vi "Bildwechsel.vi"(5 "Referenz Permanent":refnum<vi>, 7 "Referenz Mitte":refnum<vi>, 8 "nächstes Bild":T1=enum."Grafik") -> (1 "aktuelle Bildnummer":T1=enum."Grafik", 3 "VI-Referenz neu":refnum<vi>)   [LabVIEW 2020, in "Bildwechsel.lvlib"]
uses:
  Bildwechsel.lvlib
  Bild-Auswahl.ctl
  <vilib>/Utility/miscctls.llb/LVBoundsTypeDef.ctl
  VisBx Anzeige.vi
  EPA 1065/Dichtheitstest 1065-345/Konfig Leak Check.vi
  EPA 1065/Gas Analyzer Drift 1065-550/Drift Verification Konfig.vi
  EPA 1065/Interference verificaton 1065-366/VI Interference Konfig.vi
  EPA 1065/T90 1065-308/T90 Test Konfig.vi
  EPA 1065/Interference verificaton 1065-375/VI Interference Konfig.vi
  VI Anlagengrenzwerte Amium PNS.vi
  Seiten/EL3000/FID/VI FID Konfig.vi
  Seiten/EL3000/PMA/VI PMA Konfig.vi
  VI Konfiguration Kalibriergase.vi
  Seiten/Lambdasonde/VI Konfig LAMBDA.vi
  Schedule Modul/VI Schedule Seite.vi
  Seiten/System Einstellungen V2/System und Gaseinstellung V2.vi
  Seiten/CAN Konfig/VI CAN Konfig.vi
  EPA 1065/HovaCAL Interference verification/VI Interference Konfig.vi
  Allgemein/allgemeine Sub-VIs.lvlib
  Seiten/Grafik/Grafik.lvlib
  Seiten/Anlagengrenzwerte/Anlagengrenzwerte.lvlib
  Seiten/Gaszuordnung AO/Gaszuordnung AO.lvlib
  Seiten/Erweiterte Konfig/Erweiterte Konfig.lvlib
  Seiten/Anlagenuebersicht/VisBx Anzeige/Anlagenuebersicht.lvlib
  Seiten/FT-IR/FT-IR.lvlib
  PNS/PNS.lvlib
  Stoerungen/Stoerungen.lvlib
  Seiten/Statusuebersicht/Statusuebersicht.lvlib
  Seiten/EL3000/FID/FID.lvlib
  Seiten/EL3000/PMA/PMA.lvlib
  Seiten/CalGas Aufschaltung/CalGas Aufschaltung.lvlib
  Seiten/Lambdasonde/Lambda_ Komm.lvlib
  Amium PNS/Amium PNS.lvlib
  Linearisierung V2/Linearisierung v2.lvlib
  EPA 1065/Dichtheitstest 1065-345/Dichtheitstest 1065-345.lvlib
  EPA 1065/T90 1065-308/T90 Test 1065-308.lvlib
  EPA 1065/ANR Test 1065-305/ARN Test 1065-305.lvlib
  EPA 1065/Interference verificaton 1065-375/Interference verificaton 1065-375.lvlib
  EPA 1065/Interference verificaton 1065-366/Interference verificaton 1065-366.lvlib
  Schedule Modul/Schedule Modul.lvlib
  Seiten/Log Konfig/LogKonfig.lvlib
  Seiten/System Einstellungen V2/System Einstellungen V2.lvlib
  EPA 1065/Gas Analyzer Drift 1065-550/Gas Analyzer Drift 1065-550.lvlib
  Seiten/CAN Konfig/CAN Konfig.lvlib
  EPA 1065/HovaCAL Interference verification/HovaCAL Interference verificaton.lvlib
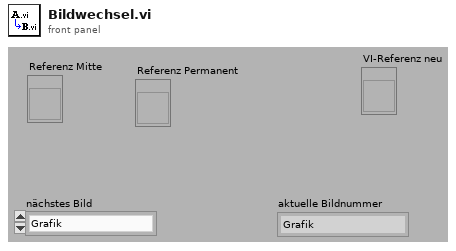
[diagram p1: front panel]
types:
  T1 = typedef "Bildwechsel.lvlib/Bild-Auswahl.ctl" = enum16{"lesen", "Initialisieren", "Beenden", "Grafik", "Anlagenübersicht", "Anlagengrenzwerte", "Log Konfig", "Gaszuordnung AO", "Erw. Konfiguration", "FT-IR  ", "Störmeldungen", "Störmeldepuffer", "Störmeldekonfig", "PNS Grenzwerte", "Statusübersicht", "Linearisierung", "ARN", "EPA Dichtheitstest", "FID", "PMA", "CalGas", "Lambda", "Interference", "Amium PNS", "EPA T90", "Interference N2O", "Scheduler", "Systemeinstellungen", "EPA Drift", "CAN Konfig", "HovaCAL Interference"}
  T2 = typedef "LVBoundsTypeDef.ctl" = cluster{"Width":u32, "Height":u32}
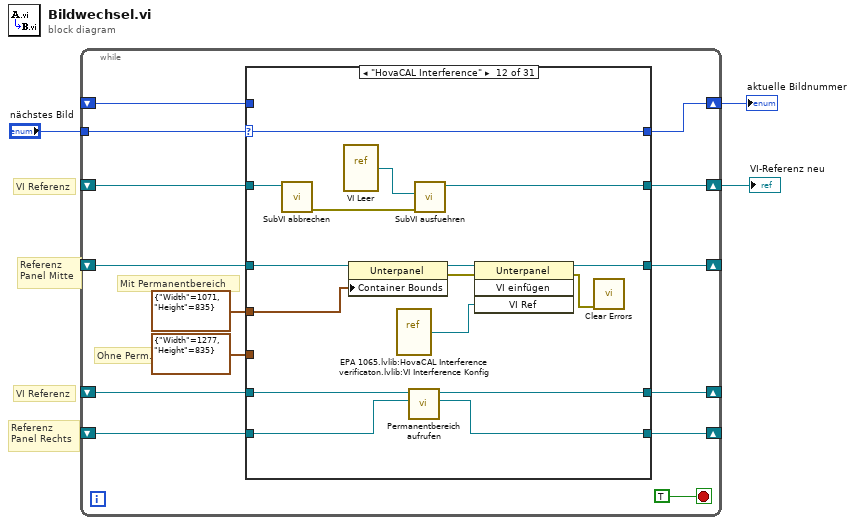
[diagram p0: block diagram]
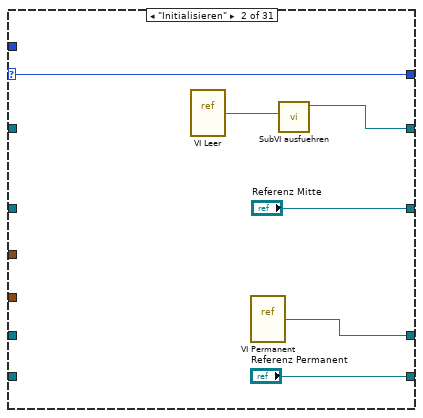
[diagram p3: hidden frame]
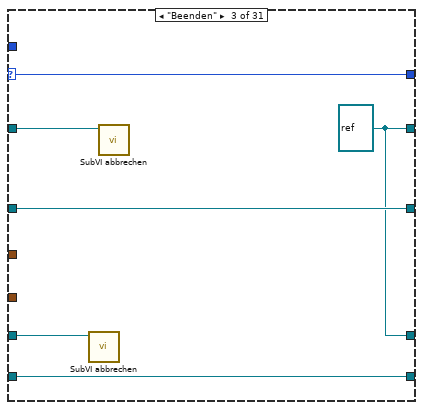
[diagram p4: hidden frame]
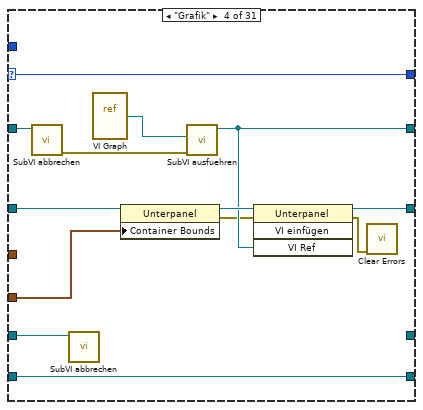
[diagram p5: hidden frame]
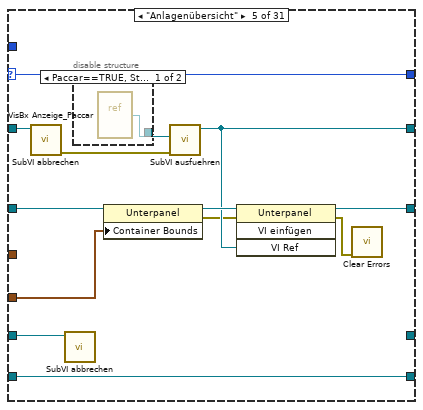
[diagram p6: hidden frame]
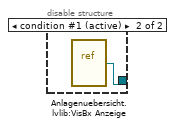
[diagram p7: hidden frame]
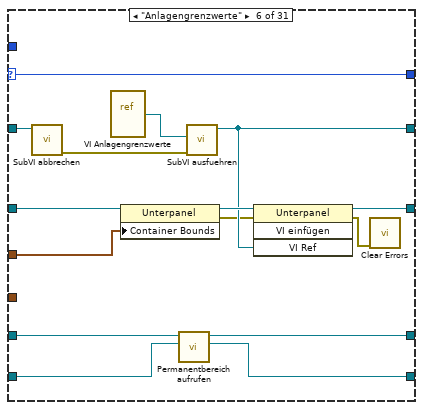
[diagram p8: hidden frame]
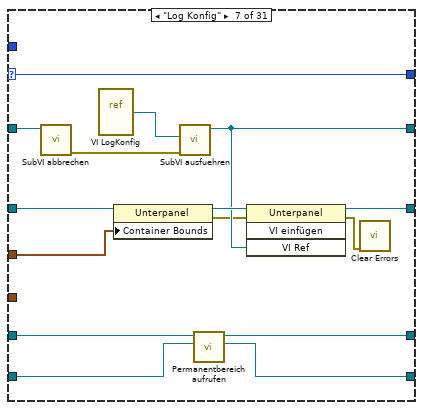
[diagram p9: hidden frame]
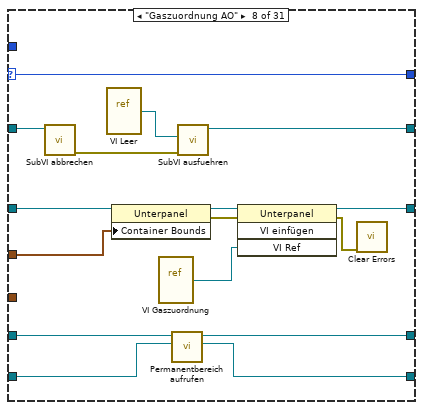
[diagram p10: hidden frame]
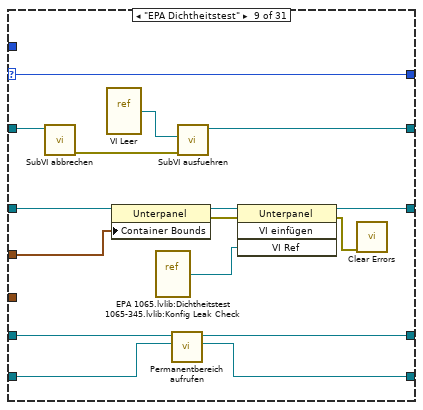
[diagram p11: hidden frame]
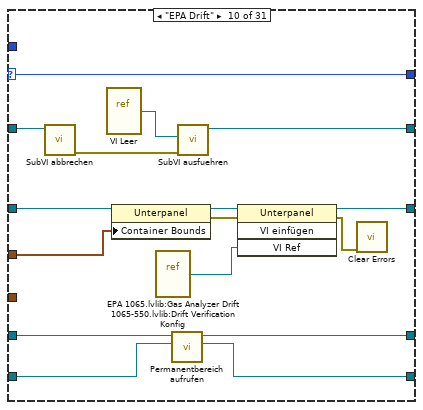
[diagram p12: hidden frame]
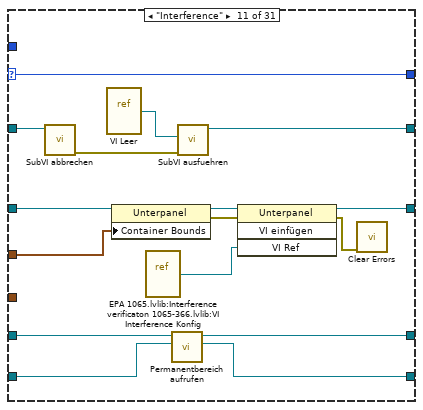
[diagram p13: hidden frame]
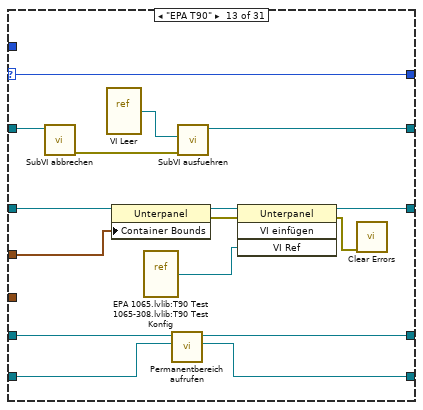
[diagram p14: hidden frame]
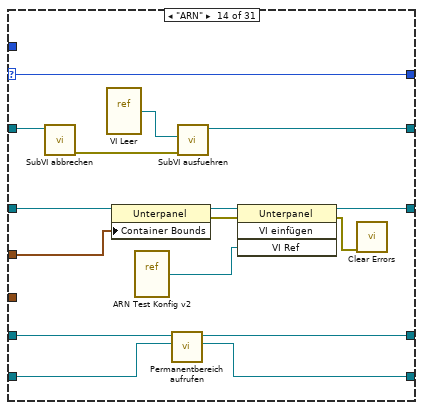
[diagram p15: hidden frame]
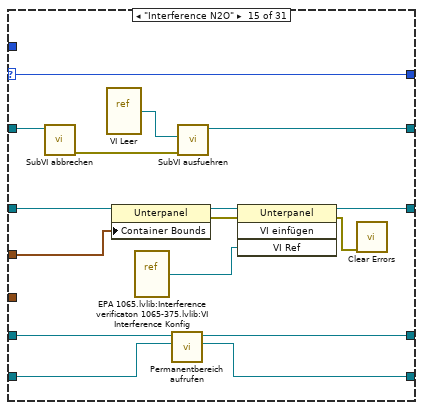
[diagram p16: hidden frame]
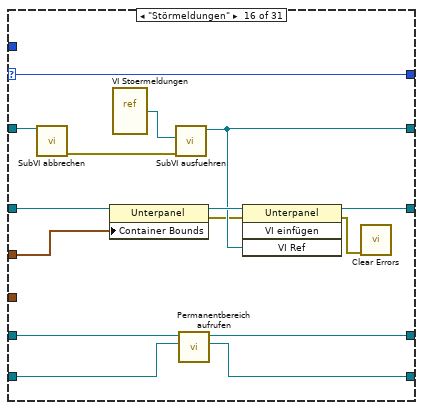
[diagram p17: hidden frame]
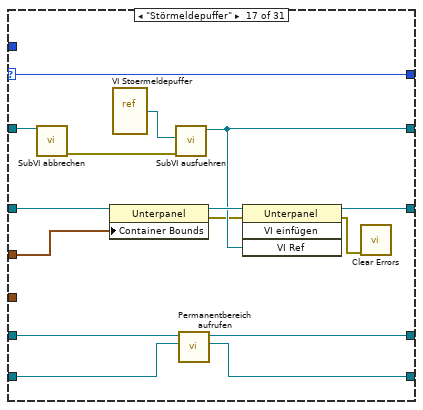
[diagram p18: hidden frame]
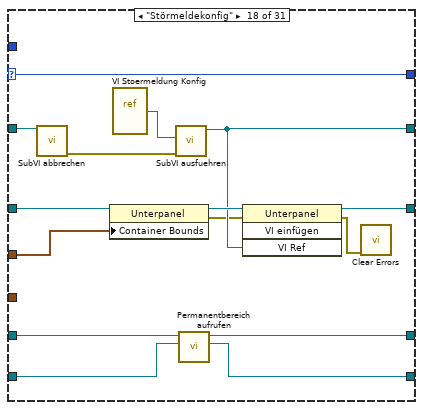
[diagram p19: hidden frame]
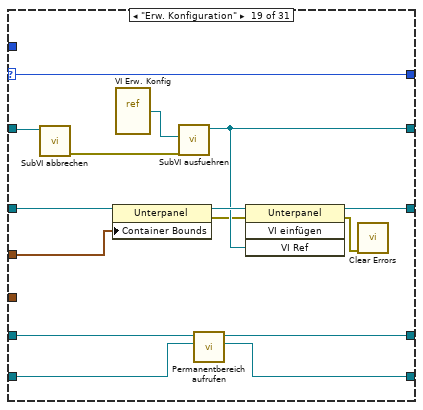
[diagram p20: hidden frame]
diagram:
  # "VI Referenz"
  # "VI Referenz"
  # "Referenz\nPanel Rechts"
  # "Referenz\nPanel Mitte"
  n1 = while {
    shift-right: [w15] -> w2
    shift-left: _ -> [w14]
    tunnel: "nächstes Bild" -> [w13]
    shift-right: [w12] -> _
    shift-left: _ -> [w11]
    shift-right: [w9] -> _
    shift-left: _ -> [w8]
    shift-right: [w7] -> w1
    shift-left: _ -> [w6]
    shift-right: [w5] -> _
    shift-left: _ -> [w4]
    stop <- TRUE stop-if-true
    # "Ohne Perm."
    # "Mit Permanentbereich"
    n2 = case shown="\"HovaCAL Interference\"" w13 {
      selector: w13 -> [_ w25 w32 w41 w53 w70 w85 w100 w117 w133 w149 w165 w181 w197 w213 w228 w243 w258 w273 w289 w304 w319 w334 w349 w364 w379 w394 w411 w427 w442 w457]
      tunnel: w14 -> [w21 _ w34 w46 w59 w76 w89 w106 w122 w138 w154 w170 w186 w202 w218 w231 w246 w261 w279 w294 w309 w324 w339 w354 w369 w384 w399 w415 w418 w433 w448]
      tunnel: [w21 w27 w31 w45 w58 w75 w91 w104 w120 w136 w152 w168 w184 w200 w216 w233 w248 w263 w278 w293 w308 w323 w338 w353 w368 w383 w398 w414 w426 w441 w456] -> w15
      tunnel: w11 -> [w20 _ w33 w44 w57 w74 w90 w107 w123 w139 w155 w171 w187 w203 w219 w232 w247 w262 w277 w292 w307 w322 w337 w352 w367 w382 w397 w413 w424 w439 w454]
      tunnel: T2 {"Width"=1071, "Height"=835} ("groß") -> [_ _ _ _ _ w73 w88 w105 w121 w137 w153 w169 w185 w201 w217 w229 w244 w259 w276 w288 w303 w318 w333 w348 w363 w378 w393 w410 w419 w434 w449]
      tunnel: T2 {"Width"=1277, "Height"=835} ("groß") -> [_ _ _ w40 w56 _ _ _ _ _ _ _ _ _ _ _ _ _ _ _ _ _ _ _ _ _ _ _ _ _ _]
      tunnel: [w20 "Referenz Mitte" w33 w42 w54 w71 w86 w103 w119 w135 w151 w167 w183 w199 w215 w230 w245 w260 w274 w290 w305 w320 w335 w350 w365 w380 w395 w412 w425 w440 w455] -> w12
      tunnel: [w19 w23 w31 _ _ w68 w81 w97 w114 w130 w146 w162 w178 w194 w210 w226 w241 w256 w269 w286 w301 w316 w331 w346 w361 w376 w391 w408 w421 w436 w451] -> w9
      tunnel: w8 -> [w19 _ w29 w39 w51 w69 w82 w98 w115 w131 w147 w163 w179 w195 w211 w227 w242 w257 w270 w287 w302 w317 w332 w347 w362 w377 w392 w409 w423 w438 w453]
      tunnel: [w22 w25 w32 w41 w53 w70 w85 w100 w117 w133 w149 w165 w181 w197 w213 w228 w243 w258 w273 w289 w304 w319 w334 w349 w364 w379 w394 w411 w427 w442 w457] -> w7
      tunnel: w6 -> [w22 _ _ _ _ _ _ _ _ _ _ _ _ _ _ _ _ _ _ _ _ _ _ _ _ _ _ _ _ _ _]
      tunnel: [w18 "Referenz Permanent" w30 w38 w50 w66 w79 w95 w112 w128 w144 w160 w176 w192 w208 w225 w240 w255 w268 w284 w299 w314 w329 w344 w359 w374 w389 w406 w420 w435 w450] -> w5
      tunnel: w4 -> [w18 _ w30 w38 w50 w67 w80 w96 w113 w129 w145 w161 w177 w193 w209 w224 w239 w254 w267 w285 w300 w315 w330 w345 w360 w375 w390 w407 w422 w437 w452]
      frame "lesen" {
      }
      frame "Initialisieren" {
        n3 = vi-ref "VI Leer.vi"() -> (w26:refnum<vi>)
        n4 = vi-ref "VI Permanent.vi"() -> (w23:refnum<vi>)
        n5 = call "SubVI ausfuehren.vi"("Referenz"=w26) -> ("vi reference"=w27:refnum<vi>)  [unwired: 10 in]
      }
      frame "Beenden" {
        w31 = refnum<vi> refnum ("vi reference")
        n6 = call "SubVI abbrechen.vi"("vi reference"=w29) -> ()  [unwired: 1 in, 6 out]
        n7 = call "SubVI abbrechen.vi"("vi reference"=w34) -> ()  [unwired: 1 in, 6 out]
      }
      frame "Grafik" {
        n8 = call "SubVI abbrechen.vi"("vi reference"=w46) -> ("error out"=w35:errorcluster)  [unwired: 1 in, 5 out]
        n9 = call "SubVI abbrechen.vi"("vi reference"=w39) -> ()  [unwired: 1 in, 6 out]
        n10 = vi-ref "VI Graph.vi"() -> (w43:refnum<vi>)
        n11 = property on="Eigenschaftsknoten" class="Unterpanel"(reference=w44, "Container Bounds"=w40) -> (reference out=w47:refnum<vi>, error out=w37:errorcluster)  [unwired: 1 in]
        n12 = call "SubVI ausfuehren.vi"("Fehler"=w35, "Referenz"=w43) -> ("vi reference"=w45:refnum<vi>)  [unwired: 9 in]
        n13 = invoke on="Methodenknoten" class="Unterpanel" method="VI einfügen"(reference=w47, error in=w37, "VI Ref"=w45) -> (reference out=w42:refnum<vi>, error out=w36:errorcluster)  [unwired: 1 in, 2 out]
        n14 = call <vilib>:"Clear Errors.vi"("error in (no error)"=w36) -> ()  [unwired: 5 in, 2 out]
      }
      frame "Anlagenübersicht" {
        n15 = call "SubVI abbrechen.vi"("vi reference"=w59) -> ("error out"=w48:errorcluster)  [unwired: 1 in, 5 out]
        n16 = call "SubVI abbrechen.vi"("vi reference"=w51) -> ()  [unwired: 1 in, 6 out]
        n17 = disable-structure shown="Paccar==TRUE, Standard" {
          disable-tunnel: [w61 w62] -> w55
          frame condition #0 {
            n18 = vi-ref "VisBx Anzeige_Paccar.vi"() -> (w61:refnum<vi>)
          }
          frame condition #1 (active) {
            n19 = vi-ref "Anlagenuebersicht.lvlib:VisBx Anzeige.vi"() -> (w62:refnum<vi>)
          }
        }
        n20 = property on="Eigenschaftsknoten" class="Unterpanel"(reference=w57, "Container Bounds"=w56) -> (reference out=w60:refnum<vi>, error out=w52:errorcluster)  [unwired: 1 in]
        n21 = call "SubVI ausfuehren.vi"("Fehler"=w48, "Referenz"=w55) -> ("vi reference"=w58:refnum<vi>)  [unwired: 9 in]
        n22 = invoke on="Methodenknoten" class="Unterpanel" method="VI einfügen"(reference=w60, error in=w52, "VI Ref"=w58) -> (reference out=w54:refnum<vi>, error out=w49:errorcluster)  [unwired: 1 in, 2 out]
        n23 = call <vilib>:"Clear Errors.vi"("error in (no error)"=w49) -> ()  [unwired: 5 in, 2 out]
      }
      frame "Anlagengrenzwerte" {
        n24 = call "SubVI abbrechen.vi"("vi reference"=w76) -> ("error out"=w63:errorcluster)  [unwired: 1 in, 5 out]
        n25 = vi-ref "VI Anlagengrenzwerte.vi"() -> (w72:refnum<vi>)
        n26 = property on="Eigenschaftsknoten" class="Unterpanel"(reference=w74, "Container Bounds"=w73) -> (reference out=w77:refnum<vi>, error out=w65:errorcluster)  [unwired: 1 in]
        n27 = call "Permanentbereich aufrufen.vi"("Permanent (Eingang)"=w67, "VI (Eingang)"=w69) -> ("Permanent (Ausgang)"=w66:refnum<vi>, "VI (Ausgang)"=w68:refnum<vi>)  [unwired: 8 in]
        n28 = call "SubVI ausfuehren.vi"("Fehler"=w63, "Referenz"=w72) -> ("vi reference"=w75:refnum<vi>)  [unwired: 9 in]
        n29 = invoke on="Methodenknoten" class="Unterpanel" method="VI einfügen"(reference=w77, error in=w65, "VI Ref"=w75) -> (reference out=w71:refnum<vi>, error out=w64:errorcluster)  [unwired: 1 in, 2 out]
        n30 = call <vilib>:"Clear Errors.vi"("error in (no error)"=w64) -> ()  [unwired: 5 in, 2 out]
      }
      frame "Log Konfig" {
        n31 = call "SubVI abbrechen.vi"("vi reference"=w89) -> ("error out"=w78:errorcluster)  [unwired: 1 in, 5 out]
        n32 = vi-ref "VI LogKonfig.vi"() -> (w87:refnum<vi>)
        n33 = property on="Eigenschaftsknoten" class="Unterpanel"(reference=w90, "Container Bounds"=w88) -> (reference out=w92:refnum<vi>, error out=w84:errorcluster)  [unwired: 1 in]
        n34 = call "SubVI ausfuehren.vi"("Fehler"=w78, "Referenz"=w87) -> ("vi reference"=w91:refnum<vi>)  [unwired: 9 in]
        n35 = call "Permanentbereich aufrufen.vi"("Permanent (Eingang)"=w80, "VI (Eingang)"=w82) -> ("Permanent (Ausgang)"=w79:refnum<vi>, "VI (Ausgang)"=w81:refnum<vi>)  [unwired: 8 in]
        n36 = invoke on="Methodenknoten" class="Unterpanel" method="VI einfügen"(reference=w92, error in=w84, "VI Ref"=w91) -> (reference out=w86:refnum<vi>, error out=w83:errorcluster)  [unwired: 1 in, 2 out]
        n37 = call <vilib>:"Clear Errors.vi"("error in (no error)"=w83) -> ()  [unwired: 5 in, 2 out]
      }
      frame "Gaszuordnung AO" {
        n38 = call "SubVI abbrechen.vi"("vi reference"=w106) -> ("error out"=w93:errorcluster)  [unwired: 1 in, 5 out]
        n39 = vi-ref "VI Leer.vi"() -> (w102:refnum<vi>)
        n40 = property on="Eigenschaftsknoten" class="Unterpanel"(reference=w107, "Container Bounds"=w105) -> (reference out=w108:refnum<vi>, error out=w94:errorcluster)  [unwired: 1 in]
        n41 = vi-ref "VI Gaszuordnung.vi"() -> (w101:refnum<vi>)
        n42 = call "Permanentbereich aufrufen.vi"("Permanent (Eingang)"=w96, "VI (Eingang)"=w98) -> ("Permanent (Ausgang)"=w95:refnum<vi>, "VI (Ausgang)"=w97:refnum<vi>)  [unwired: 8 in]
        n43 = call "SubVI ausfuehren.vi"("Fehler"=w93, "Referenz"=w102) -> ("vi reference"=w104:refnum<vi>)  [unwired: 9 in]
        n44 = invoke on="Methodenknoten" class="Unterpanel" method="VI einfügen"(reference=w108, error in=w94, "VI Ref"=w101) -> (reference out=w103:refnum<vi>, error out=w99:errorcluster)  [unwired: 1 in, 2 out]
        n45 = call <vilib>:"Clear Errors.vi"("error in (no error)"=w99) -> ()  [unwired: 5 in, 2 out]
      }
      frame "EPA Dichtheitstest" {
        n46 = call "SubVI abbrechen.vi"("vi reference"=w122) -> ("error out"=w110:errorcluster)  [unwired: 1 in, 5 out]
        n47 = vi-ref "VI Leer.vi"() -> (w118:refnum<vi>)
        n48 = property on="Eigenschaftsknoten" class="Unterpanel"(reference=w123, "Container Bounds"=w121) -> (reference out=w124:refnum<vi>, error out=w111:errorcluster)  [unwired: 1 in]
        n49 = vi-ref "EPA 1065.lvlib:Dichtheitstest 1065-345.lvlib:Konfig Leak Check.vi"() -> (w109:refnum<vi>)
        n50 = call "Permanentbereich aufrufen.vi"("Permanent (Eingang)"=w113, "VI (Eingang)"=w115) -> ("Permanent (Ausgang)"=w112:refnum<vi>, "VI (Ausgang)"=w114:refnum<vi>)  [unwired: 8 in]
        n51 = call "SubVI ausfuehren.vi"("Fehler"=w110, "Referenz"=w118) -> ("vi reference"=w120:refnum<vi>)  [unwired: 9 in]
        n52 = invoke on="Methodenknoten" class="Unterpanel" method="VI einfügen"(reference=w124, error in=w111, "VI Ref"=w109) -> (reference out=w119:refnum<vi>, error out=w116:errorcluster)  [unwired: 1 in, 2 out]
        n53 = call <vilib>:"Clear Errors.vi"("error in (no error)"=w116) -> ()  [unwired: 5 in, 2 out]
      }
      frame "EPA Drift" {
        n54 = call "SubVI abbrechen.vi"("vi reference"=w138) -> ("error out"=w126:errorcluster)  [unwired: 1 in, 5 out]
        n55 = vi-ref "VI Leer.vi"() -> (w134:refnum<vi>)
        n56 = property on="Eigenschaftsknoten" class="Unterpanel"(reference=w139, "Container Bounds"=w137) -> (reference out=w140:refnum<vi>, error out=w127:errorcluster)  [unwired: 1 in]
        n57 = vi-ref "EPA 1065.lvlib:Gas Analyzer Drift 1065-550.lvlib:Drift Verification Konfig.vi"() -> (w125:refnum<vi>)
        n58 = call "Permanentbereich aufrufen.vi"("Permanent (Eingang)"=w129, "VI (Eingang)"=w131) -> ("Permanent (Ausgang)"=w128:refnum<vi>, "VI (Ausgang)"=w130:refnum<vi>)  [unwired: 8 in]
        n59 = call "SubVI ausfuehren.vi"("Fehler"=w126, "Referenz"=w134) -> ("vi reference"=w136:refnum<vi>)  [unwired: 9 in]
        n60 = invoke on="Methodenknoten" class="Unterpanel" method="VI einfügen"(reference=w140, error in=w127, "VI Ref"=w125) -> (reference out=w135:refnum<vi>, error out=w132:errorcluster)  [unwired: 1 in, 2 out]
        n61 = call <vilib>:"Clear Errors.vi"("error in (no error)"=w132) -> ()  [unwired: 5 in, 2 out]
      }
      frame "Interference" {
        n62 = call "SubVI abbrechen.vi"("vi reference"=w154) -> ("error out"=w142:errorcluster)  [unwired: 1 in, 5 out]
        n63 = vi-ref "VI Leer.vi"() -> (w150:refnum<vi>)
        n64 = property on="Eigenschaftsknoten" class="Unterpanel"(reference=w155, "Container Bounds"=w153) -> (reference out=w156:refnum<vi>, error out=w143:errorcluster)  [unwired: 1 in]
        n65 = vi-ref "EPA 1065.lvlib:Interference verificaton 1065-366.lvlib:VI Interference Konfig.vi"() -> (w141:refnum<vi>)
        n66 = call "Permanentbereich aufrufen.vi"("Permanent (Eingang)"=w145, "VI (Eingang)"=w147) -> ("Permanent (Ausgang)"=w144:refnum<vi>, "VI (Ausgang)"=w146:refnum<vi>)  [unwired: 8 in]
        n67 = call "SubVI ausfuehren.vi"("Fehler"=w142, "Referenz"=w150) -> ("vi reference"=w152:refnum<vi>)  [unwired: 9 in]
        n68 = invoke on="Methodenknoten" class="Unterpanel" method="VI einfügen"(reference=w156, error in=w143, "VI Ref"=w141) -> (reference out=w151:refnum<vi>, error out=w148:errorcluster)  [unwired: 1 in, 2 out]
        n69 = call <vilib>:"Clear Errors.vi"("error in (no error)"=w148) -> ()  [unwired: 5 in, 2 out]
      }
      frame "HovaCAL Interference" {
        n70 = call "SubVI abbrechen.vi"("vi reference"=w170) -> ("error out"=w158:errorcluster)  [unwired: 1 in, 5 out]
        n71 = vi-ref "VI Leer.vi"() -> (w166:refnum<vi>)
        n72 = property on="Eigenschaftsknoten" class="Unterpanel"(reference=w171, "Container Bounds"=w169) -> (reference out=w172:refnum<vi>, error out=w159:errorcluster)  [unwired: 1 in]
        n73 = vi-ref "EPA 1065.lvlib:HovaCAL Interference verificaton.lvlib:VI Interference Konfig.vi"() -> (w157:refnum<vi>)
        n74 = call "Permanentbereich aufrufen.vi"("Permanent (Eingang)"=w161, "VI (Eingang)"=w163) -> ("Permanent (Ausgang)"=w160:refnum<vi>, "VI (Ausgang)"=w162:refnum<vi>)  [unwired: 8 in]
        n75 = call "SubVI ausfuehren.vi"("Fehler"=w158, "Referenz"=w166) -> ("vi reference"=w168:refnum<vi>)  [unwired: 9 in]
        n76 = invoke on="Methodenknoten" class="Unterpanel" method="VI einfügen"(reference=w172, error in=w159, "VI Ref"=w157) -> (reference out=w167:refnum<vi>, error out=w164:errorcluster)  [unwired: 1 in, 2 out]
        n77 = call <vilib>:"Clear Errors.vi"("error in (no error)"=w164) -> ()  [unwired: 5 in, 2 out]
      }
      frame "EPA T90" {
        n78 = call "SubVI abbrechen.vi"("vi reference"=w186) -> ("error out"=w174:errorcluster)  [unwired: 1 in, 5 out]
        n79 = vi-ref "VI Leer.vi"() -> (w182:refnum<vi>)
        n80 = property on="Eigenschaftsknoten" class="Unterpanel"(reference=w187, "Container Bounds"=w185) -> (reference out=w188:refnum<vi>, error out=w175:errorcluster)  [unwired: 1 in]
        n81 = vi-ref "EPA 1065.lvlib:T90 Test 1065-308.lvlib:T90 Test Konfig.vi"() -> (w173:refnum<vi>)
        n82 = call "Permanentbereich aufrufen.vi"("Permanent (Eingang)"=w177, "VI (Eingang)"=w179) -> ("Permanent (Ausgang)"=w176:refnum<vi>, "VI (Ausgang)"=w178:refnum<vi>)  [unwired: 8 in]
        n83 = call "SubVI ausfuehren.vi"("Fehler"=w174, "Referenz"=w182) -> ("vi reference"=w184:refnum<vi>)  [unwired: 9 in]
        n84 = invoke on="Methodenknoten" class="Unterpanel" method="VI einfügen"(reference=w188, error in=w175, "VI Ref"=w173) -> (reference out=w183:refnum<vi>, error out=w180:errorcluster)  [unwired: 1 in, 2 out]
        n85 = call <vilib>:"Clear Errors.vi"("error in (no error)"=w180) -> ()  [unwired: 5 in, 2 out]
      }
      frame "ARN" {
        n86 = call "SubVI abbrechen.vi"("vi reference"=w202) -> ("error out"=w190:errorcluster)  [unwired: 1 in, 5 out]
        n87 = vi-ref "VI Leer.vi"() -> (w198:refnum<vi>)
        n88 = property on="Eigenschaftsknoten" class="Unterpanel"(reference=w203, "Container Bounds"=w201) -> (reference out=w204:refnum<vi>, error out=w191:errorcluster)  [unwired: 1 in]
        n89 = vi-ref "ARN Test Konfig v2.vi"() -> (w189:refnum<vi>)
        n90 = call "Permanentbereich aufrufen.vi"("Permanent (Eingang)"=w193, "VI (Eingang)"=w195) -> ("Permanent (Ausgang)"=w192:refnum<vi>, "VI (Ausgang)"=w194:refnum<vi>)  [unwired: 8 in]
        n91 = call "SubVI ausfuehren.vi"("Fehler"=w190, "Referenz"=w198) -> ("vi reference"=w200:refnum<vi>)  [unwired: 9 in]
        n92 = invoke on="Methodenknoten" class="Unterpanel" method="VI einfügen"(reference=w204, error in=w191, "VI Ref"=w189) -> (reference out=w199:refnum<vi>, error out=w196:errorcluster)  [unwired: 1 in, 2 out]
        n93 = call <vilib>:"Clear Errors.vi"("error in (no error)"=w196) -> ()  [unwired: 5 in, 2 out]
      }
      frame "Interference N2O" {
        n94 = call "SubVI abbrechen.vi"("vi reference"=w218) -> ("error out"=w206:errorcluster)  [unwired: 1 in, 5 out]
        n95 = vi-ref "VI Leer.vi"() -> (w214:refnum<vi>)
        n96 = property on="Eigenschaftsknoten" class="Unterpanel"(reference=w219, "Container Bounds"=w217) -> (reference out=w220:refnum<vi>, error out=w207:errorcluster)  [unwired: 1 in]
        n97 = vi-ref "EPA 1065.lvlib:Interference verificaton 1065-375.lvlib:VI Interference Konfig.vi"() -> (w205:refnum<vi>)
        n98 = call "Permanentbereich aufrufen.vi"("Permanent (Eingang)"=w209, "VI (Eingang)"=w211) -> ("Permanent (Ausgang)"=w208:refnum<vi>, "VI (Ausgang)"=w210:refnum<vi>)  [unwired: 8 in]
        n99 = call "SubVI ausfuehren.vi"("Fehler"=w206, "Referenz"=w214) -> ("vi reference"=w216:refnum<vi>)  [unwired: 9 in]
        n100 = invoke on="Methodenknoten" class="Unterpanel" method="VI einfügen"(reference=w220, error in=w207, "VI Ref"=w205) -> (reference out=w215:refnum<vi>, error out=w212:errorcluster)  [unwired: 1 in, 2 out]
        n101 = call <vilib>:"Clear Errors.vi"("error in (no error)"=w212) -> ()  [unwired: 5 in, 2 out]
      }
      frame "Störmeldungen" {
        n102 = call "SubVI abbrechen.vi"("vi reference"=w231) -> ("error out"=w221:errorcluster)  [unwired: 1 in, 5 out]
        n103 = property on="Eigenschaftsknoten" class="Unterpanel"(reference=w232, "Container Bounds"=w229) -> (reference out=w235:refnum<vi>, error out=w223:errorcluster)  [unwired: 1 in]
        n104 = vi-ref "VI Stoermeldungen.vi"() -> (w234:refnum<vi>)
        n105 = call "SubVI ausfuehren.vi"("Fehler"=w221, "Referenz"=w234) -> ("vi reference"=w233:refnum<vi>)  [unwired: 9 in]
        n106 = call "Permanentbereich aufrufen.vi"("Permanent (Eingang)"=w224, "VI (Eingang)"=w227) -> ("Permanent (Ausgang)"=w225:refnum<vi>, "VI (Ausgang)"=w226:refnum<vi>)  [unwired: 8 in]
        n107 = invoke on="Methodenknoten" class="Unterpanel" method="VI einfügen"(reference=w235, error in=w223, "VI Ref"=w233) -> (reference out=w230:refnum<vi>, error out=w222:errorcluster)  [unwired: 1 in, 2 out]
        n108 = call <vilib>:"Clear Errors.vi"("error in (no error)"=w222) -> ()  [unwired: 5 in, 2 out]
      }
      frame "Störmeldepuffer" {
        n109 = call "SubVI abbrechen.vi"("vi reference"=w246) -> ("error out"=w236:errorcluster)  [unwired: 1 in, 5 out]
        n110 = property on="Eigenschaftsknoten" class="Unterpanel"(reference=w247, "Container Bounds"=w244) -> (reference out=w250:refnum<vi>, error out=w238:errorcluster)  [unwired: 1 in]
        n111 = vi-ref "VI Stoermeldepuffer.vi"() -> (w249:refnum<vi>)
        n112 = call "SubVI ausfuehren.vi"("Fehler"=w236, "Referenz"=w249) -> ("vi reference"=w248:refnum<vi>)  [unwired: 9 in]
        n113 = call "Permanentbereich aufrufen.vi"("Permanent (Eingang)"=w239, "VI (Eingang)"=w242) -> ("Permanent (Ausgang)"=w240:refnum<vi>, "VI (Ausgang)"=w241:refnum<vi>)  [unwired: 8 in]
        n114 = invoke on="Methodenknoten" class="Unterpanel" method="VI einfügen"(reference=w250, error in=w238, "VI Ref"=w248) -> (reference out=w245:refnum<vi>, error out=w237:errorcluster)  [unwired: 1 in, 2 out]
        n115 = call <vilib>:"Clear Errors.vi"("error in (no error)"=w237) -> ()  [unwired: 5 in, 2 out]
      }
      frame "Störmeldekonfig" {
        n116 = call "SubVI abbrechen.vi"("vi reference"=w261) -> ("error out"=w251:errorcluster)  [unwired: 1 in, 5 out]
        n117 = property on="Eigenschaftsknoten" class="Unterpanel"(reference=w262, "Container Bounds"=w259) -> (reference out=w265:refnum<vi>, error out=w253:errorcluster)  [unwired: 1 in]
        n118 = vi-ref "VI Stoermeldung Konfig.vi"() -> (w264:refnum<vi>)
        n119 = call "SubVI ausfuehren.vi"("Fehler"=w251, "Referenz"=w264) -> ("vi reference"=w263:refnum<vi>)  [unwired: 9 in]
        n120 = call "Permanentbereich aufrufen.vi"("Permanent (Eingang)"=w254, "VI (Eingang)"=w257) -> ("Permanent (Ausgang)"=w255:refnum<vi>, "VI (Ausgang)"=w256:refnum<vi>)  [unwired: 8 in]
        n121 = invoke on="Methodenknoten" class="Unterpanel" method="VI einfügen"(reference=w265, error in=w253, "VI Ref"=w263) -> (reference out=w260:refnum<vi>, error out=w252:errorcluster)  [unwired: 1 in, 2 out]
        n122 = call <vilib>:"Clear Errors.vi"("error in (no error)"=w252) -> ()  [unwired: 5 in, 2 out]
      }
      frame "Erw. Konfiguration" {
        n123 = call "SubVI abbrechen.vi"("vi reference"=w279) -> ("error out"=w266:errorcluster)  [unwired: 1 in, 5 out]
        n124 = property on="Eigenschaftsknoten" class="Unterpanel"(reference=w277, "Container Bounds"=w276) -> (reference out=w280:refnum<vi>, error out=w272:errorcluster)  [unwired: 1 in]
        n125 = vi-ref "VI Erw. Konfig.vi"() -> (w275:refnum<vi>)
        n126 = call "SubVI ausfuehren.vi"("Fehler"=w266, "Referenz"=w275) -> ("vi reference"=w278:refnum<vi>)  [unwired: 9 in]
        n127 = call "Permanentbereich aufrufen.vi"("Permanent (Eingang)"=w267, "VI (Eingang)"=w270) -> ("Permanent (Ausgang)"=w268:refnum<vi>, "VI (Ausgang)"=w269:refnum<vi>)  [unwired: 8 in]
        n128 = invoke on="Methodenknoten" class="Unterpanel" method="VI einfügen"(reference=w280, error in=w272, "VI Ref"=w278) -> (reference out=w274:refnum<vi>, error out=w271:errorcluster)  [unwired: 1 in, 2 out]
        n129 = call <vilib>:"Clear Errors.vi"("error in (no error)"=w271) -> ()  [unwired: 5 in, 2 out]
      }
      frame "FT-IR  " {
        n130 = call "SubVI abbrechen.vi"("vi reference"=w294) -> ("error out"=w281:errorcluster)  [unwired: 1 in, 5 out]
        n131 = vi-ref "VI Konfig FT-IR.vi"() -> (w291:refnum<vi>)
        n132 = property on="Eigenschaftsknoten" class="Unterpanel"(reference=w292, "Container Bounds"=w288) -> (reference out=w295:refnum<vi>, error out=w283:errorcluster)  [unwired: 1 in]
        n133 = call "Permanentbereich aufrufen.vi"("Permanent (Eingang)"=w285, "VI (Eingang)"=w287) -> ("Permanent (Ausgang)"=w284:refnum<vi>, "VI (Ausgang)"=w286:refnum<vi>)  [unwired: 8 in]
        n134 = call "SubVI ausfuehren.vi"("Fehler"=w281, "Referenz"=w291) -> ("vi reference"=w293:refnum<vi>)  [unwired: 9 in]
        n135 = invoke on="Methodenknoten" class="Unterpanel" method="VI einfügen"(reference=w295, error in=w283, "VI Ref"=w293) -> (reference out=w290:refnum<vi>, error out=w282:errorcluster)  [unwired: 1 in, 2 out]
        n136 = call <vilib>:"Clear Errors.vi"("error in (no error)"=w282) -> ()  [unwired: 5 in, 2 out]
      }
      frame "PNS Grenzwerte" {
        n137 = call "SubVI abbrechen.vi"("vi reference"=w309) -> ("error out"=w296:errorcluster)  [unwired: 1 in, 5 out]
        n138 = vi-ref "VI Anlagengrenzwerte PNS.vi"() -> (w306:refnum<vi>)
        n139 = property on="Eigenschaftsknoten" class="Unterpanel"(reference=w307, "Container Bounds"=w303) -> (reference out=w310:refnum<vi>, error out=w298:errorcluster)  [unwired: 1 in]
        n140 = call "Permanentbereich aufrufen.vi"("Permanent (Eingang)"=w300, "VI (Eingang)"=w302) -> ("Permanent (Ausgang)"=w299:refnum<vi>, "VI (Ausgang)"=w301:refnum<vi>)  [unwired: 8 in]
        n141 = call "SubVI ausfuehren.vi"("Fehler"=w296, "Referenz"=w306) -> ("vi reference"=w308:refnum<vi>)  [unwired: 9 in]
        n142 = invoke on="Methodenknoten" class="Unterpanel" method="VI einfügen"(reference=w310, error in=w298, "VI Ref"=w308) -> (reference out=w305:refnum<vi>, error out=w297:errorcluster)  [unwired: 1 in, 2 out]
        n143 = call <vilib>:"Clear Errors.vi"("error in (no error)"=w297) -> ()  [unwired: 5 in, 2 out]
      }
      frame "Amium PNS" {
        n144 = call "SubVI abbrechen.vi"("vi reference"=w324) -> ("error out"=w311:errorcluster)  [unwired: 1 in, 5 out]
        n145 = vi-ref "Amium PNS.lvlib:VI Anlagengrenzwerte Amium PNS.vi"() -> (w321:refnum<vi>)
        n146 = property on="Eigenschaftsknoten" class="Unterpanel"(reference=w322, "Container Bounds"=w318) -> (reference out=w325:refnum<vi>, error out=w313:errorcluster)  [unwired: 1 in]
        n147 = call "Permanentbereich aufrufen.vi"("Permanent (Eingang)"=w315, "VI (Eingang)"=w317) -> ("Permanent (Ausgang)"=w314:refnum<vi>, "VI (Ausgang)"=w316:refnum<vi>)  [unwired: 8 in]
        n148 = call "SubVI ausfuehren.vi"("Fehler"=w311, "Referenz"=w321) -> ("vi reference"=w323:refnum<vi>)  [unwired: 9 in]
        n149 = invoke on="Methodenknoten" class="Unterpanel" method="VI einfügen"(reference=w325, error in=w313, "VI Ref"=w323) -> (reference out=w320:refnum<vi>, error out=w312:errorcluster)  [unwired: 1 in, 2 out]
        n150 = call <vilib>:"Clear Errors.vi"("error in (no error)"=w312) -> ()  [unwired: 5 in, 2 out]
      }
      frame "Statusübersicht" {
        n151 = call "SubVI abbrechen.vi"("vi reference"=w339) -> ("error out"=w326:errorcluster)  [unwired: 1 in, 5 out]
        n152 = vi-ref "VI Statusuebersicht.vi"() -> (w336:refnum<vi>)
        n153 = property on="Eigenschaftsknoten" class="Unterpanel"(reference=w337, "Container Bounds"=w333) -> (reference out=w340:refnum<vi>, error out=w328:errorcluster)  [unwired: 1 in]
        n154 = call "Permanentbereich aufrufen.vi"("Permanent (Eingang)"=w330, "VI (Eingang)"=w332) -> ("Permanent (Ausgang)"=w329:refnum<vi>, "VI (Ausgang)"=w331:refnum<vi>)  [unwired: 8 in]
        n155 = call "SubVI ausfuehren.vi"("Fehler"=w326, "Referenz"=w336) -> ("vi reference"=w338:refnum<vi>)  [unwired: 9 in]
        n156 = invoke on="Methodenknoten" class="Unterpanel" method="VI einfügen"(reference=w340, error in=w328, "VI Ref"=w338) -> (reference out=w335:refnum<vi>, error out=w327:errorcluster)  [unwired: 1 in, 2 out]
        n157 = call <vilib>:"Clear Errors.vi"("error in (no error)"=w327) -> ()  [unwired: 5 in, 2 out]
      }
      frame "FID" {
        n158 = call "SubVI abbrechen.vi"("vi reference"=w354) -> ("error out"=w341:errorcluster)  [unwired: 1 in, 5 out]
        n159 = vi-ref "ABB-EL3000.lvlib:FID.lvlib:VI FID Konfig.vi"() -> (w351:refnum<vi>)
        n160 = property on="Eigenschaftsknoten" class="Unterpanel"(reference=w352, "Container Bounds"=w348) -> (reference out=w355:refnum<vi>, error out=w343:errorcluster)  [unwired: 1 in]
        n161 = call "Permanentbereich aufrufen.vi"("Permanent (Eingang)"=w345, "VI (Eingang)"=w347) -> ("Permanent (Ausgang)"=w344:refnum<vi>, "VI (Ausgang)"=w346:refnum<vi>)  [unwired: 8 in]
        n162 = call "SubVI ausfuehren.vi"("Fehler"=w341, "Referenz"=w351) -> ("vi reference"=w353:refnum<vi>)  [unwired: 9 in]
        n163 = invoke on="Methodenknoten" class="Unterpanel" method="VI einfügen"(reference=w355, error in=w343, "VI Ref"=w353) -> (reference out=w350:refnum<vi>, error out=w342:errorcluster)  [unwired: 1 in, 2 out]
        n164 = call <vilib>:"Clear Errors.vi"("error in (no error)"=w342) -> ()  [unwired: 5 in, 2 out]
      }
      frame "PMA" {
        n165 = call "SubVI abbrechen.vi"("vi reference"=w369) -> ("error out"=w356:errorcluster)  [unwired: 1 in, 5 out]
        n166 = vi-ref "ABB-EL3000.lvlib:PMA.lvlib:VI PMA Konfig.vi"() -> (w366:refnum<vi>)
        n167 = property on="Eigenschaftsknoten" class="Unterpanel"(reference=w367, "Container Bounds"=w363) -> (reference out=w370:refnum<vi>, error out=w358:errorcluster)  [unwired: 1 in]
        n168 = call "Permanentbereich aufrufen.vi"("Permanent (Eingang)"=w360, "VI (Eingang)"=w362) -> ("Permanent (Ausgang)"=w359:refnum<vi>, "VI (Ausgang)"=w361:refnum<vi>)  [unwired: 8 in]
        n169 = call "SubVI ausfuehren.vi"("Fehler"=w356, "Referenz"=w366) -> ("vi reference"=w368:refnum<vi>)  [unwired: 9 in]
        n170 = invoke on="Methodenknoten" class="Unterpanel" method="VI einfügen"(reference=w370, error in=w358, "VI Ref"=w368) -> (reference out=w365:refnum<vi>, error out=w357:errorcluster)  [unwired: 1 in, 2 out]
        n171 = call <vilib>:"Clear Errors.vi"("error in (no error)"=w357) -> ()  [unwired: 5 in, 2 out]
      }
      frame "CalGas" {
        n172 = call "SubVI abbrechen.vi"("vi reference"=w384) -> ("error out"=w371:errorcluster)  [unwired: 1 in, 5 out]
        n173 = vi-ref "CalGas Aufschaltung.lvlib:VI Konfiguration Kalibriergase.vi"() -> (w381:refnum<vi>)
        n174 = property on="Eigenschaftsknoten" class="Unterpanel"(reference=w382, "Container Bounds"=w378) -> (reference out=w385:refnum<vi>, error out=w373:errorcluster)  [unwired: 1 in]
        n175 = call "Permanentbereich aufrufen.vi"("Permanent (Eingang)"=w375, "VI (Eingang)"=w377) -> ("Permanent (Ausgang)"=w374:refnum<vi>, "VI (Ausgang)"=w376:refnum<vi>)  [unwired: 8 in]
        n176 = call "SubVI ausfuehren.vi"("Fehler"=w371, "Referenz"=w381) -> ("vi reference"=w383:refnum<vi>)  [unwired: 9 in]
        n177 = invoke on="Methodenknoten" class="Unterpanel" method="VI einfügen"(reference=w385, error in=w373, "VI Ref"=w383) -> (reference out=w380:refnum<vi>, error out=w372:errorcluster)  [unwired: 1 in, 2 out]
        n178 = call <vilib>:"Clear Errors.vi"("error in (no error)"=w372) -> ()  [unwired: 5 in, 2 out]
      }
      frame "Lambda" {
        n179 = call "SubVI abbrechen.vi"("vi reference"=w399) -> ("error out"=w386:errorcluster)  [unwired: 1 in, 5 out]
        n180 = vi-ref "Lambda_ Komm.lvlib:VI Konfig LAMBDA.vi"() -> (w396:refnum<vi>)
        n181 = property on="Eigenschaftsknoten" class="Unterpanel"(reference=w397, "Container Bounds"=w393) -> (reference out=w400:refnum<vi>, error out=w388:errorcluster)  [unwired: 1 in]
        n182 = call "Permanentbereich aufrufen.vi"("Permanent (Eingang)"=w390, "VI (Eingang)"=w392) -> ("Permanent (Ausgang)"=w389:refnum<vi>, "VI (Ausgang)"=w391:refnum<vi>)  [unwired: 8 in]
        n183 = call "SubVI ausfuehren.vi"("Fehler"=w386, "Referenz"=w396) -> ("vi reference"=w398:refnum<vi>)  [unwired: 9 in]
        n184 = invoke on="Methodenknoten" class="Unterpanel" method="VI einfügen"(reference=w400, error in=w388, "VI Ref"=w398) -> (reference out=w395:refnum<vi>, error out=w387:errorcluster)  [unwired: 1 in, 2 out]
        n185 = call <vilib>:"Clear Errors.vi"("error in (no error)"=w387) -> ()  [unwired: 5 in, 2 out]
      }
      frame "Linearisierung" {
        # "#Option10xSpanAuto"
        n186 = call "SubVI abbrechen.vi"("vi reference"=w415) -> ("error out"=w403:errorcluster)  [unwired: 1 in, 5 out]
        n187 = vi-ref "VI Leer.vi"() -> (w401:refnum<vi>)
        n188 = property on="Eigenschaftsknoten" class="Unterpanel"(reference=w413, "Container Bounds"=w410) -> (reference out=w416:refnum<vi>, error out=w405:errorcluster)  [unwired: 1 in]
        n189 = vi-ref "VI Linearisierung v2.vi"() -> (w402:refnum<vi>)
        n190 = call "Permanentbereich aufrufen.vi"("Permanent (Eingang)"=w407, "VI (Eingang)"=w409) -> ("Permanent (Ausgang)"=w406:refnum<vi>, "VI (Ausgang)"=w408:refnum<vi>)  [unwired: 8 in]
        n191 = call "SubVI ausfuehren.vi"("Fehler"=w403, "Referenz"=w401) -> ("vi reference"=w414:refnum<vi>)  [unwired: 9 in]
        n192 = invoke on="Methodenknoten" class="Unterpanel" method="VI einfügen"(reference=w416, error in=w405, "VI Ref"=w402) -> (reference out=w412:refnum<vi>, error out=w404:errorcluster)  [unwired: 1 in, 2 out]
        n193 = call <vilib>:"Clear Errors.vi"("error in (no error)"=w404) -> ()  [unwired: 5 in, 2 out]
      }
      frame "Scheduler" {
        n194 = call "SubVI abbrechen.vi"("vi reference"=w418) -> ("error out"=w428:errorcluster)  [unwired: 1 in, 5 out]
        n195 = vi-ref "Schedule Modul.lvlib:VI Schedule Seite.vi"() -> (w430:refnum<vi>)
        n196 = property on="Eigenschaftsknoten" class="Unterpanel"(reference=w424, "Container Bounds"=w419) -> (reference out=w431:refnum<vi>, error out=w429:errorcluster)  [unwired: 1 in]
        n197 = call "Permanentbereich aufrufen.vi"("Permanent (Eingang)"=w422, "VI (Eingang)"=w423) -> ("Permanent (Ausgang)"=w420:refnum<vi>, "VI (Ausgang)"=w421:refnum<vi>)  [unwired: 8 in]
        n198 = call "SubVI ausfuehren.vi"("Fehler"=w428, "Referenz"=w430) -> ("vi reference"=w426:refnum<vi>)  [unwired: 9 in]
        n199 = invoke on="Methodenknoten" class="Unterpanel" method="VI einfügen"(reference=w431, error in=w429, "VI Ref"=w426) -> (reference out=w425:refnum<vi>, error out=w417:errorcluster)  [unwired: 1 in, 2 out]
        n200 = call <vilib>:"Clear Errors.vi"("error in (no error)"=w417) -> ()  [unwired: 5 in, 2 out]
      }
      frame "Systemeinstellungen" {
        n201 = call "SubVI abbrechen.vi"("vi reference"=w433) -> ("error out"=w443:errorcluster)  [unwired: 1 in, 5 out]
        n202 = vi-ref "System Einstellungen V2.lvlib:System und Gaseinstellung V2.vi"() -> (w445:refnum<vi>)
        n203 = property on="Eigenschaftsknoten" class="Unterpanel"(reference=w439, "Container Bounds"=w434) -> (reference out=w446:refnum<vi>, error out=w444:errorcluster)  [unwired: 1 in]
        n204 = call "Permanentbereich aufrufen.vi"("Permanent (Eingang)"=w437, "VI (Eingang)"=w438) -> ("Permanent (Ausgang)"=w435:refnum<vi>, "VI (Ausgang)"=w436:refnum<vi>)  [unwired: 8 in]
        n205 = call "SubVI ausfuehren.vi"("Fehler"=w443, "Referenz"=w445) -> ("vi reference"=w441:refnum<vi>)  [unwired: 9 in]
        n206 = invoke on="Methodenknoten" class="Unterpanel" method="VI einfügen"(reference=w446, error in=w444, "VI Ref"=w441) -> (reference out=w440:refnum<vi>, error out=w432:errorcluster)  [unwired: 1 in, 2 out]
        n207 = call <vilib>:"Clear Errors.vi"("error in (no error)"=w432) -> ()  [unwired: 5 in, 2 out]
      }
      frame "CAN Konfig" {
        n208 = call "SubVI abbrechen.vi"("vi reference"=w448) -> ("error out"=w458:errorcluster)  [unwired: 1 in, 5 out]
        n209 = vi-ref "CAN Konfig.lvlib:VI CAN Konfig.vi"() -> (w460:refnum<vi>)
        n210 = property on="Eigenschaftsknoten" class="Unterpanel"(reference=w454, "Container Bounds"=w449) -> (reference out=w461:refnum<vi>, error out=w459:errorcluster)  [unwired: 1 in]
        n211 = call "Permanentbereich aufrufen.vi"("Permanent (Eingang)"=w452, "VI (Eingang)"=w453) -> ("Permanent (Ausgang)"=w450:refnum<vi>, "VI (Ausgang)"=w451:refnum<vi>)  [unwired: 8 in]
        n212 = call "SubVI ausfuehren.vi"("Fehler"=w458, "Referenz"=w460) -> ("vi reference"=w456:refnum<vi>)  [unwired: 9 in]
        n213 = invoke on="Methodenknoten" class="Unterpanel" method="VI einfügen"(reference=w461, error in=w459, "VI Ref"=w456) -> (reference out=w455:refnum<vi>, error out=w447:errorcluster)  [unwired: 1 in, 2 out]
        n214 = call <vilib>:"Clear Errors.vi"("error in (no error)"=w447) -> ()  [unwired: 5 in, 2 out]
      }
    }
  }
  "VI-Referenz neu" <- w2
  "aktuelle Bildnummer" <- w1
